vi "创建蜂鸟对象.vi"() -> (3 "Hummingbird.lvclass":refnum<class "Hummingbird.lvclass">)   [LabVIEW 2020, in "Hummingbird.lvclass"]
uses:
  Hummingbird.lvclass
  Animal/Animal.lvclass/Animal.ctl
  Animal/Animal.lvclass
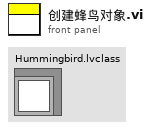
[diagram p1: front panel]
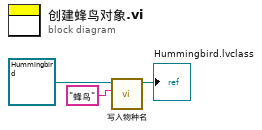
[diagram p0: block diagram]
diagram:
  n1 = call "写入物种名.vi"("物种名"="蜂鸟", "Animal输入"=refnum<class "Hummingbird.lvclass"> refnum ("Hummingbird.lvclass")) -> ("Animal输出"=→"Hummingbird.lvclass":refnum<class "Hummingbird.lvclass">)  [unwired: 8 in, 1 out]
